vi "GET_ALL.vi"(8 "error in (no error)":errorcluster, 11 "Instrument in":refnum<class "Instrument.lvclass">) -> (0 "error out":errorcluster, 2 "getAll":variant, 3 "Instrument out":refnum<class "Instrument.lvclass">)   [LabVIEW 2016, in "Instrument.lvclass"]
uses:
  Instrument.lvclass
  Typedefs/Instrument.Commands--Enum.ctl
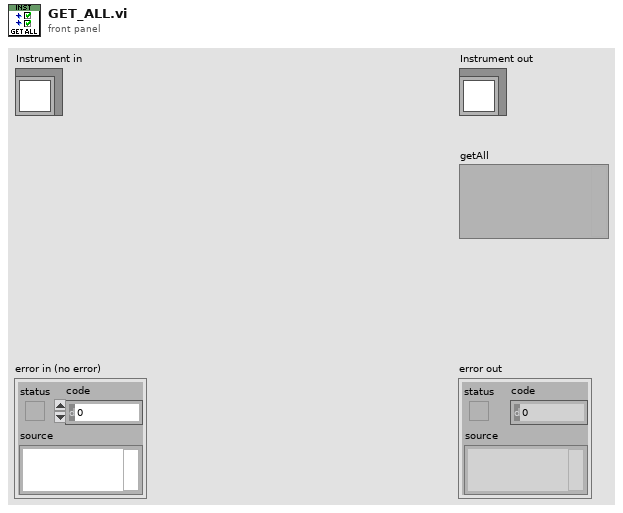
[diagram p1: front panel]
types:
  T1 = typedef "Instrument.lvclass/Instrument.Commands--Enum.ctl" = enum16{"HELP", "ACK", "getAll"}
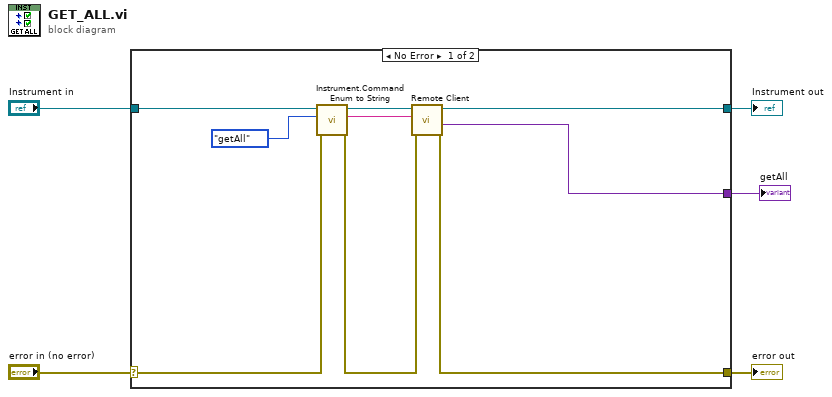
[diagram p0: block diagram]
diagram:
  n1 = case shown="No Error" "error in (no error)" {
    selector: "error in (no error)" -> [w8 w16]
    tunnel: [w14 w16] -> w4
    tunnel: [w13 w15] -> w2
    tunnel: "Instrument in" -> [w10 w15]
    tunnel: [w12 _] -> w1
    frame No Error {
      n2 = call "Instrument.Command Enum to String.vi"("error in (no error)"=w8, "Commands"=Instrument.Commands--Enum."getAll", "Instrument in"=w10) -> ("error out"=w7:errorcluster, "Command"=w11:string, "Instrument out"=w9:refnum<class "Instrument.lvclass">)  [unwired: 5 in, 1 out]
      n3 = call "Remote Client.vi"("error in (no error)"=w7, "Command"=w11, "Instrument in"=w9) -> ("error out"=w14:errorcluster, "Data out"=w12:variant, "Instrument out"=w13:refnum<class "Instrument.lvclass">)  [unwired: 5 in, 1 out]
    }
    frame Error {
    }
  }
  "error out" <- w4
  "Instrument out" <- w2
  "getAll" <- w1
